vi "Conf Offset.vi"(11 "Offset in":sgl[][](array[numeric])) -> (3 "Offset Out":sgl[][](array[numeric]))   [LabVIEW 2014, in "MSX-E3711.lvlib" / "MSX-E3711.lvclass"]
doc: "Configuro el offset con los valores que cargue el usuario o con los que traiga por defecto el programa."
uses:
  MSX-E3711Class/MSX-E3711.lvclass
panel:
  in  "Cancelar":bool
  in  "Save Button":bool
  # "Offset Configuration"
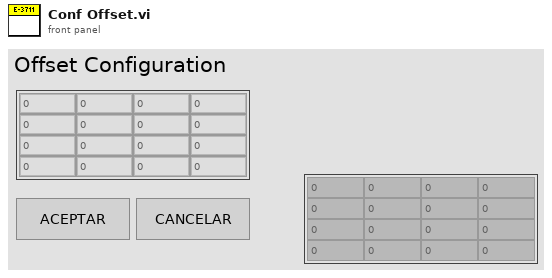
[diagram p1: front panel]
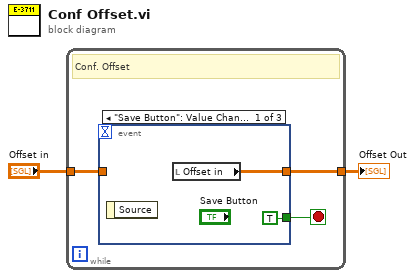
[diagram p0: block diagram]
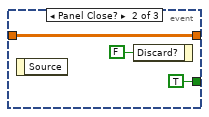
[diagram p2: hidden frame]
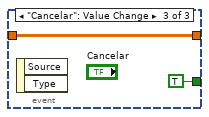
[diagram p3: hidden frame]
diagram:
  n1 = while {
    tunnel: [w4] -> w1
    tunnel: "Offset in" -> [w3]
    stop <- w5 stop-if-true
    # "Conf. Offset"
    n2 = event shown="[0] \"Save Button\": Value Change" {
      selector: _ -> [_ _ _]
      dyn-events: _ -> [_ _ _]
      timeout: _ -> [_ _ _]
      tunnel: [TRUE ("Save Button") TRUE ("Save Button") TRUE ("Save Button")] -> w5
      tunnel: [w7 w8 w11] -> w4
      tunnel: w3 -> [_ w8 w11]
      event "Save Button": Value Change {
        n3 = event-data() -> ()  [unwired: 1 in, 1 out]
        n4 = local read "Offset in"() -> (w7:sgl[][])
      }
      event Panel Close? {
        n5 = event-data() -> ()  [unwired: 1 in, 1 out]
        n6 = event-data("Discard?"=FALSE) -> ()  [unwired: 1 in, 1 out]
      }
      event "Cancelar": Value Change {
        n7 = event-data() -> ()  [unwired: 1 in, 2 out]
      }
    }
  }
  "Offset Out" <- w1
